vi "RVC 2-link serial robot 2.vi"() -> ()   [LabVIEW 2014]
uses:
  <vilib>/Analysis/Matrix/Datatypes/RealMatrix.ctl
  <vilib>/robotics/Kinematics/DH Kinematic Parameters.ctl
  <vilib>/robotics/Kinematics/Link/Joint Type.ctl
  <vilib>/robotics/Kinematics/Analytical/Initialize Generic Serial Arm.vi
  <vilib>/robotics/Kinematics/Analytical/NI_Robotics_AnalyticKinematics.lvlib
  <vilib>/robotics/Kinematics/Robot/NI_Robotics_Serial Robot Arm.lvclass
  <vilib>/Analysis/Matrix/NI_Matrix.lvlib
  <vilib>/robotics/Kinematics/Link/NI_Robotics_Link.lvclass
panel:
  out "Array":T1[](array[typedef])
  in  "joint positions":dbl[](array[numeric])=[0.0, 0.0]
  out "transformation":picture
  out "forward kinematics":T3
  out "3D Picture":refnum<vi>(3d-picture)
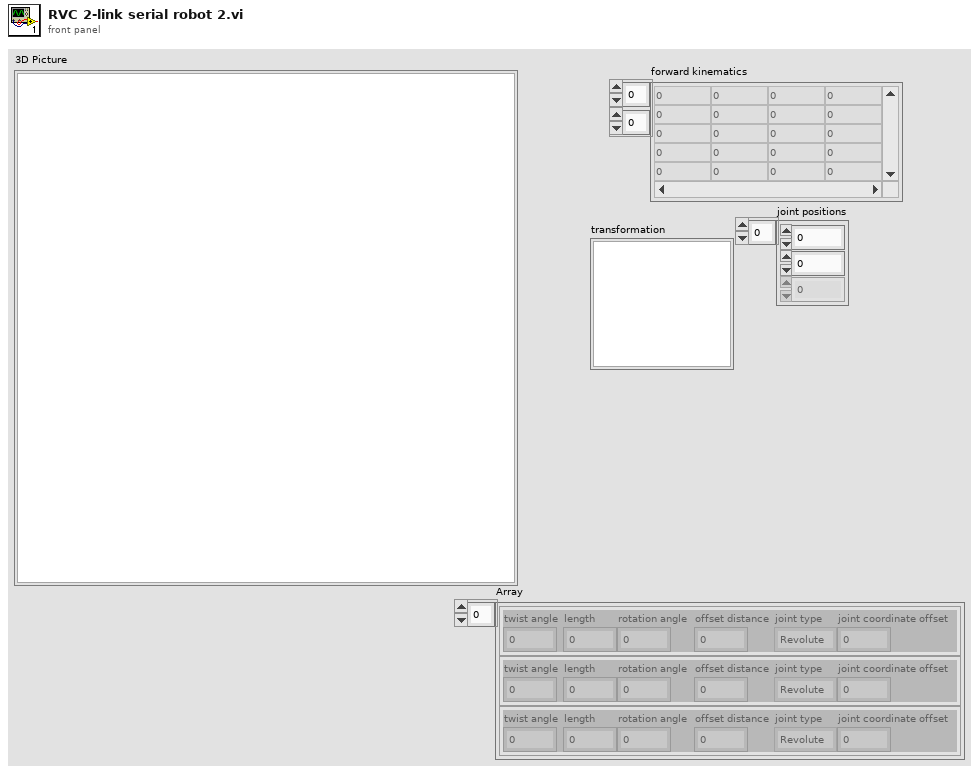
[diagram p1: front panel]
types:
  T1 = typedef "DH Kinematic Parameters.ctl" = cluster{"twist angle":dbl, "length":dbl, "rotation angle":dbl, "offset distance":dbl, "joint type":T2, "joint coordinate offset":dbl}
  T2 = typedef "NI_Robotics_Link.lvclass/Joint Type.ctl" = enum16{"Revolute", "Prismatic"}
  T3 = typedef "NI_Matrix.lvlib/RealMatrix.ctl" = dbl[][]
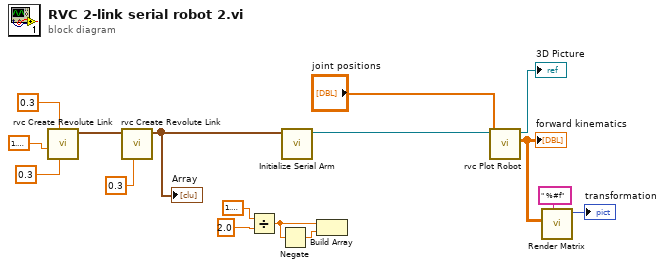
[diagram p0: block diagram]
diagram:
  n1 = call "rvc Create Revolute Link.vi"("length (a)"=0.3, "offset distance (d)"=0.3, "twist angle (alpha)"=1.5707963267948966) -> ("Array"=w10:T1[])  [unwired: 8 in]
  n2 = call "rvc Create Revolute Link.vi"("length (a)"=0.3, "Array 2"=w10) -> ("Array"=w16:T1[])  [unwired: 9 in]
  "Array" <- w16
  n3 = Divide(x=1.5707963267948966, y=2.0) -> (x/y=w12:dbl)
  n4 = Negate(x=w12) -> (-x=w11:dbl)
  n5 = call-poly <vilib>:"Initialize Serial Arm.vi"("kinematic parameters"=w16) -> ("serial arm out"=w2:refnum<class "NI_Robotics_Serial Robot Arm.lvclass">)  [unwired: 9 in, 1 out]
  n6 = Build Array(w12, w11) -> ()  [unwired: 1 out]
  n7 = call "rvc Plot Robot.vi"("joint positions"="joint positions", "NI_Robotics_Serial Robot Arm in"=w2) -> ("forward kinematics"=w5:T3, "Scene Object Out"=→"3D Picture":refnum<vi>)  [unwired: 7 in, 1 out]
  "forward kinematics" <- w5
  n8 = call "Render Matrix.vi"("format string"=" %#f", "A"=w5) -> ("picture out"=→"transformation":picture)  [unwired: 9 in]
